vi "LV4.vi"() -> ()   [LabVIEW 2014]
uses:
  <vilib>/Utility/file.llb/Read From Spreadsheet File (string).vi
  <vilib>/Utility/file.llb/Write To Spreadsheet File (string).vi
panel:
  out "text":string
  out "all rows":string[][](array[string])
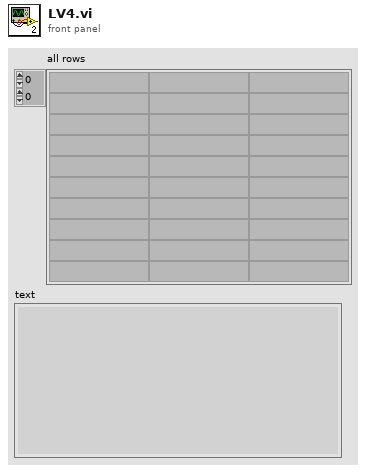
[diagram p1: front panel]
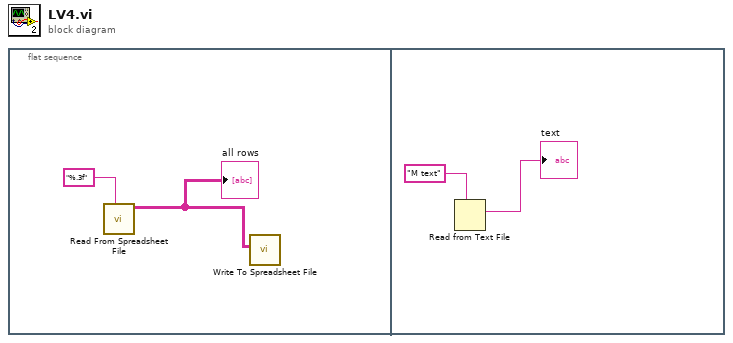
[diagram p0: block diagram]
diagram:
  n1 = flat-sequence {
    frame #0 {
      n2 = call-poly <vilib>:"Read From Spreadsheet File.vi"("format (%s)"="%.3f" ("format (%.3f)")) -> ("all rows"=w1:string[][])  [unwired: 6 in, 4 out]
      "all rows" <- w1
      n3 = call-poly <vilib>:"Write To Spreadsheet File.vi"("2D data"=w1) -> ()  [unwired: 7 in, 1 out]
    }
    frame #1 {
      n4 = Read from Text File(prompt (Open existing file)="M text") -> (text=→"text":string)  [unwired: 3 in, 3 out]
    }
  }
